vi "Read Attributes.vi"(11 "Connected Msg":refnum<class "Connected Msg.lvclass">) -> (2 "Payload":T1)   [LabVIEW 2020, in "Legacy Nested Endpoint.lvlib" / "Connected Msg.lvclass"]
uses:
  Connected Msg.lvclass
  <vilib>/ActorFramework/Message Enqueuer/Message Enqueuer.lvclass
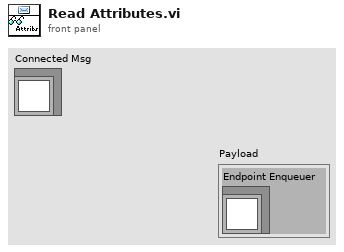
[diagram p1: front panel]
types:
  T1 = cluster{"Endpoint Enqueuer":refnum<class "Message Enqueuer.lvclass">}
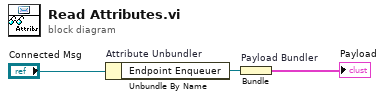
[diagram p0: block diagram]
diagram:
  n1 = Unbundle By Name "Attribute Unbundler"("Connected Msg") -> ("Endpoint Enqueuer"=w1:refnum<class "Message Enqueuer.lvclass">)
  n2 = Bundle "Payload Bundler"("Endpoint Enqueuer"=w1) -> (→"Payload":T1)  [unwired: 1 in]
